vi "SearchAndReplaceStd.vi"(4 "continue capture index":i32, 5 "replace capture index":i32, 6 "offset":i32, 7 "replace all (F)":bool, 8 "error in":errorcluster, 9 "replace to":string, 10 "search pattern":string, 11 "string":string) -> (0 "error out":errorcluster, 1 "offset past replacement":i32, 2 "number of replacements":i32, 3 "result string":string)   [LabVIEW 2021, in "libpcre2-8.lvlib"]
uses:
  libpcre2-8.lvlib
  Pcre2MoOfSubstrNumFmOv.vi
  Pcre2CompileError.vi
  Pcre2ErrorNull.vi
  Pcre2LibError.vi
  Pcre2FnkCallError.vi
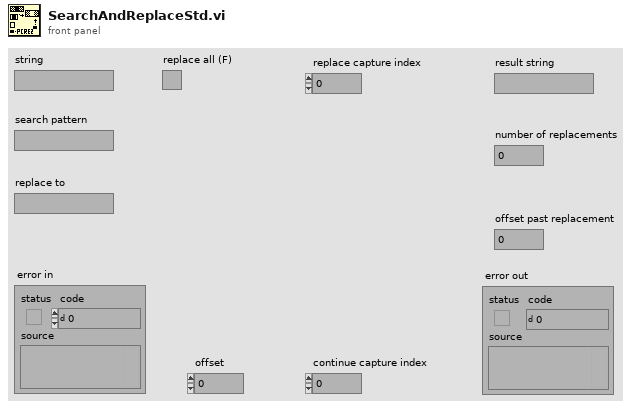
[diagram p1: front panel]
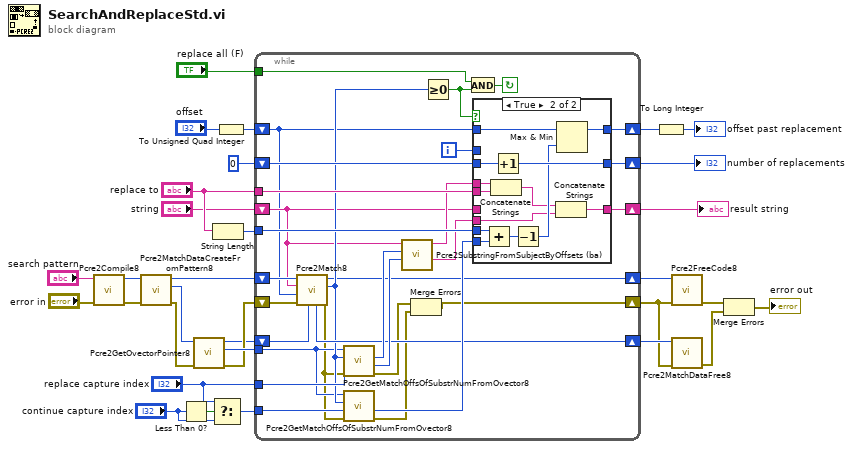
[diagram p0: block diagram]
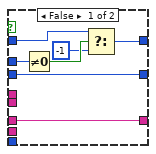
[diagram p2: hidden frame]
diagram:
  n1 = call "Pcre2Compile8.vi"("error in"="error in", "Pattern"="search pattern") -> ("error out"=w5:errorcluster, "pCode"=w6:u64)  [unwired: 8 in]
  n2 = call "Pcre2MatchDataCreateFromPattern8.vi"("error in"=w5, "pCode"=w6) -> ("error out"=w22:errorcluster, "pMatchData"=w24:u64, "pCode"=w26:u64)  [unwired: 7 in]
  n3 = Less Than 0?(x="continue capture index") -> (x < 0?=w30:bool)
  n4 = call "Pcre2GetOvectorPointer8.vi"("error in"=w22, "pMatchData"=w24) -> ("error out"=w21:errorcluster, "pOvector"=w23:u64, "pMatchData"=w20:u64)  [unwired: 7 in]
  n5 = Select(t="replace capture index", s=w30, f="continue capture index") -> (s? t:f=w31:i32)
  n6 = String Length(string="replace to") -> (length=w29:i32)
  n7 = To Unsigned Quad Integer(1:"offset") -> (0:w25:u64)
  n8 = while {
    shift-right: [w39] -> w18
    shift-left: w26 -> [w51]
    shift-right: [w32] -> w17
    shift-left: w21 -> [w50]
    shift-right: [w58] -> w13
    shift-left: w25 -> [w35]
    shift-right: [w60] -> w14
    shift-left: "string" -> [w36]
    shift-right: [w55] -> w12
    shift-left: 0 -> [w56]
    tunnel: "replace all (F)" -> [w54]
    tunnel: "replace to" -> [w53]
    tunnel: w29 -> [w52]
    tunnel: w31 -> [w43]
    tunnel: w23 -> [w38]
    tunnel: "replace capture index" -> [w48]
    shift-right: [w41] -> w19
    shift-left: w20 -> [w49]
    i -> [w57]
    stop <- w61 continue-if-true
    n9 = call "Pcre2Match8.vi"("pMatchData"=w49, "error in"=w50, "StartOffset"=w35, "Subject"=w36, "pCode"=w51) -> ("error out"=w37:errorcluster, "MatchResult"=w40:i32, "pCode"=w39:u64, "pMatchData"=w41:u64)  [unwired: 3 in]
    n10 = call "Pcre2GetMatchOffsOfSubstrNumFromOvector8.vi"("error in"=w37, "Number"=w48, "MatchResult"=w40, "pOvector"=w38) -> ("error out"=w34:errorcluster, "OffsetPastMatch"=w46:i32, "MatchOffset"=w47:i32)  [unwired: 4 in, 1 out]
    n11 = call "Pcre2GetMatchOffsOfSubstrNumFromOvector8.vi"("error in"=w37, "Number"=w43, "MatchResult"=w40, "pOvector"=w38) -> ("error out"=w33:errorcluster, "OffsetPastMatch"=w42:i32)  [unwired: 4 in, 2 out]
    n12 = call "Pcre2SubstringFromSubjectByOffsets (ba).vi"("OffsetPastMatch"=w46, "MatchOffset"=w47, "Subject"=w36) -> ("AfterSubstring"=w44:string, "BeforeSubstring"=w45:string)  [unwired: 7 in]
    n13 = Merge Errors(w34, w33) -> (w32:errorcluster)
    n14 = Greater Or Equal To 0?(x=w40) -> (x >= 0?=w59:bool)
    n15 = And(x=w54, y=w59) -> (x .and. y?=w61:bool)
    n16 = case shown="True" w59 {
      tunnel: w45 -> [_ w81]
      tunnel: w44 -> [_ w69]
      tunnel: [w68 w80] -> w60
      tunnel: w36 -> [w68 _]
      tunnel: [w67 w76] -> w58
      tunnel: w57 -> [w65 _]
      tunnel: w35 -> [w64 w77]
      tunnel: w56 -> [w62 w79]
      tunnel: [w62 w78] -> w55
      tunnel: w53 -> [_ w75]
      tunnel: w42 -> [_ w72]
      tunnel: w52 -> [_ w74]
      frame False {
        n17 = Not Equal To 0?(x=w65) -> (x != 0?=w66:bool)
        n18 = Select(t=w64, s=w66, f=-1) -> (s? t:f=w67:u64)
      }
      frame True {
        n19 = Add(x=w74, y=w72) -> (x+y=w73:i32)
        n20 = Concatenate Strings(w81, w75) -> (w70:string)
        n21 = Increment(x=w79) -> (x+1=w78:i32)
        n22 = Decrement(x=w73) -> (x-1=w71:i32)
        n23 = Concatenate Strings(w70, w69) -> (w80:string)
        n24 = Max & Min(x=w77, y=w71) -> (max(x,y)=w76:u64)  [unwired: 1 out]
      }
    }
  }
  "result string" <- w14
  "number of replacements" <- w12
  n25 = To Long Integer(number=w13) -> (32bit integer=→"offset past replacement":i32)
  n26 = call "Pcre2FreeCode8.vi"("error in"=w17, "pCode"=w18) -> ("error out"=w4:errorcluster)  [unwired: 9 in]
  n27 = call "Pcre2MatchDataFree8.vi"("error in"=w17, "pMatchData"=w19) -> ("error out"=w3:errorcluster)  [unwired: 9 in]
  n28 = Merge Errors(w4, w3) -> (→"error out":errorcluster)
